vi "Lakeshore 331 Apply Settings.vi"(8 "error in (no error)":errorcluster, 11 "Lakeshore 331 in":refnum<class "Lakeshore 331.lvclass">) -> (0 "error out":errorcluster, 3 "Lakeshore 331 out":refnum<class "Lakeshore 331.lvclass">)   [LabVIEW 2022 SP3, in "Lakeshore 331.lvclass"]
uses:
  Lakeshore 331.lvclass
  Lakeshore 331.lvclass/Lakeshore 331.ctl
  <instrlib>/Lake Shore Cryotronics 331/Lake Shore Cryotronics 331.lvlib
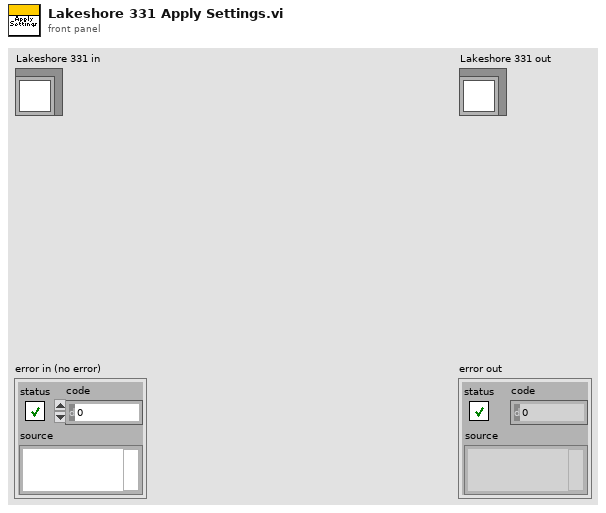
[diagram p1: front panel]
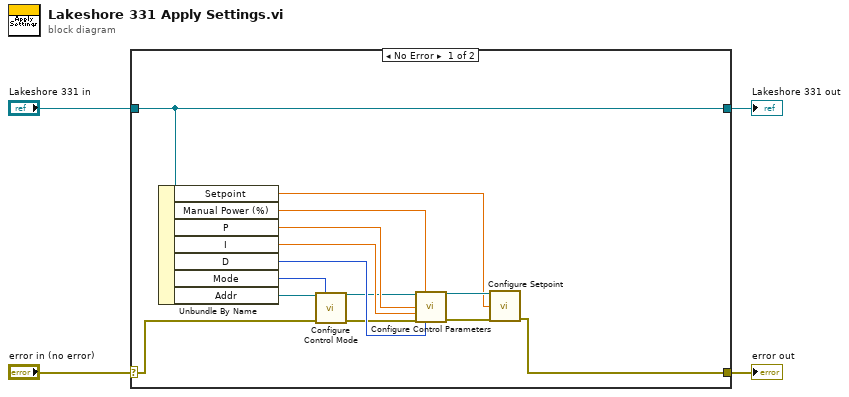
[diagram p0: block diagram]
diagram:
  n1 = case shown="No Error" "error in (no error)" {
    selector: "error in (no error)" -> [w10 w20]
    tunnel: [w5 w20] -> w3
    tunnel: [w15 w19] -> w1
    tunnel: "Lakeshore 331 in" -> [w15 w19]
    frame No Error {
      n2 = Unbundle By Name(w15) -> ("Setpoint"=w6:dbl, "Manual Power (%)"=w14:dbl, "P"=w18:dbl, "I"=w17:dbl, "D"=w16:u16, "Mode"=w9:u16, "Addr"=w13:refnum<visa-resource-name>)
      n3 = call <instrlib>:"Configure Control Mode.vi"("VISA resource name"=w13, "Control Mode (0: Manual PID)"=w9, "error in (no error)"=w10) -> ("VISA resource name out"=w11:refnum<visa-resource-name>, "error out"=w12:errorcluster)  [unwired: 11 in]
      n4 = call <instrlib>:"Configure Control Parameters.vi"("VISA resource name"=w11, "Manual Output (0.000 %)"=w14, "Gain (P) (0.0)"=w18, "Reset (I) (0.0)"=w17, "error in (no error)"=w12, "Rate (D) (0)"=w16) -> ("VISA resource name out"=w7:refnum<visa-resource-name>, "error out"=w8:errorcluster)  [unwired: 8 in]
      n5 = call <instrlib>:"Configure Setpoint.vi"("VISA resource name"=w7, "Setpoint (0.0000)"=w6, "error in (no error)"=w8) -> ("error out"=w5:errorcluster)  [unwired: 11 in, 1 out]
    }
    frame Error {
    }
  }
  "error out" <- w3
  "Lakeshore 331 out" <- w1
